vi "CAPTH-IPC-Quit Analysis.vi"(0 "IPC":T1, 11 "error in (no error)":errorcluster) -> (15 "error out":errorcluster)   [LabVIEW 2020]
uses:
  Typedefs/CAPTH-IPC.ctl
  Typedefs/CAPTH-Start Data.ctl
  Typedefs/CAPTH-Parameters.ctl
  Typedefs/CAPTH-Stimulus.ctl
  Typedefs/CAPTH-Response.ctl
  Typedefs/CAPTH-Analysis Message.ctl
  Typedefs/CAPTH-Analysis Action.ctl
  Typedefs/CAPTH-StimCon.ctl
  Typedefs/CAPTH-Analysis Data Properties.ctl
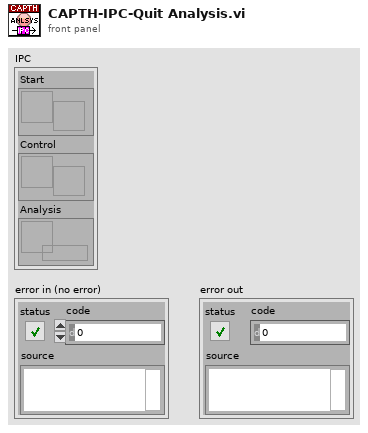
[diagram p1: front panel]
types:
  T1 = typedef "CAPTH-IPC.ctl" = cluster{"Start":refnum<notifier>, "Control":refnum<notifier>, "Analysis":refnum<queue>}
  T2 = typedef "CAPTH-Analysis Action.ctl" = enum16{"Init", "Raw", "Avg", "Quit"}
  T3 = typedef "CAPTH-Analysis Message.ctl" = cluster{"Action":T2, "Data":dbl[], "StimCon":T4, "Properties":T5, "Num":i32}
  T4 = typedef "CAPTH-StimCon.ctl" = cluster{"ear":i32, "freq":i32, "Max SPL":dbl}
  T5 = typedef "CAPTH-Analysis Data Properties.ctl" = cluster{"atten":dbl, "amp":dbl, "1dB":bool}
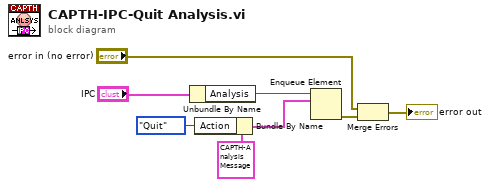
[diagram p0: block diagram]
diagram:
  n1 = Unbundle By Name("IPC") -> ("Analysis"=w6:refnum<queue>)
  n2 = Bundle By Name(cluster=T3 {"Action"=enum."Init", "Data"=[], "StimCon"={"ear"=0, "freq"=0, "Max SPL"=0.0}, "Properties"={"atten"=0.0, "amp"=0.0, "1dB"=FALSE}, "Num"=0} ("Message"), "Action"=CAPTH-Analysis_Action."Quit") -> (w7:T3)
  n3 = Enqueue Element(queue=w6, element=w7) -> (error out=w8:errorcluster)  [unwired: 2 in, 2 out]
  n4 = Merge Errors("error in (no error)", w8) -> (→"error out":errorcluster)
